vi "Пwiczenie 1.vi"() -> ()   [LabVIEW 2017]
panel:
  in  "Czyœæ":bool
  out "Aktualny wynik":dbl format="%#.1f"
  in  "Czêstotliwoœæ próbkowania":u16(ring) items=["1 Hz"=1, "2 Hz"=2, "5 Hz"=5, "10 Hz"=10]
  in  "Okres":dbl(knob) step=2.0 scale=0.0..60.0
  in  "Amplituda":dbl(knob) step=1.0 scale=0.0..100.0
  in  "Czas narastania":dbl(knob) step=1.0 scale=0.0..60.0
  in  "Amplituda":dbl(knob) step=1.0 scale=0.0..100.0
  in  "Max":dbl(knob) step=1.0 scale=0.0..100.0
  in  "Min":dbl(knob) max=30.0 step=1.0 scale=0.0..100.0
  out "Wynik":dbl(graph)
  in  "STOP":bool
  in  "Tryb pracy":i32(knob) scale=1.0..3.0
  # "TRYB 1 - WARTOŒCI LOSOWE"
  # "TRYB 2 - SYGNA£ PI£OKSZTA£TNY"
  # "TRYB  3 - SYGNA£ TRÓJK¥TNY"
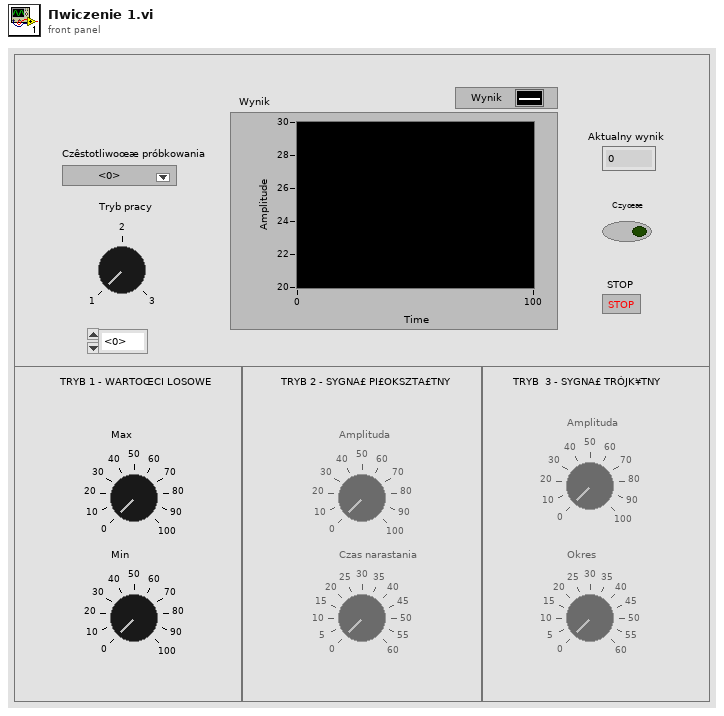
[diagram p1: front panel]
types:
  T1 = enum8{"Enabled", "Disabled", "Disabled and Grayed Out"}
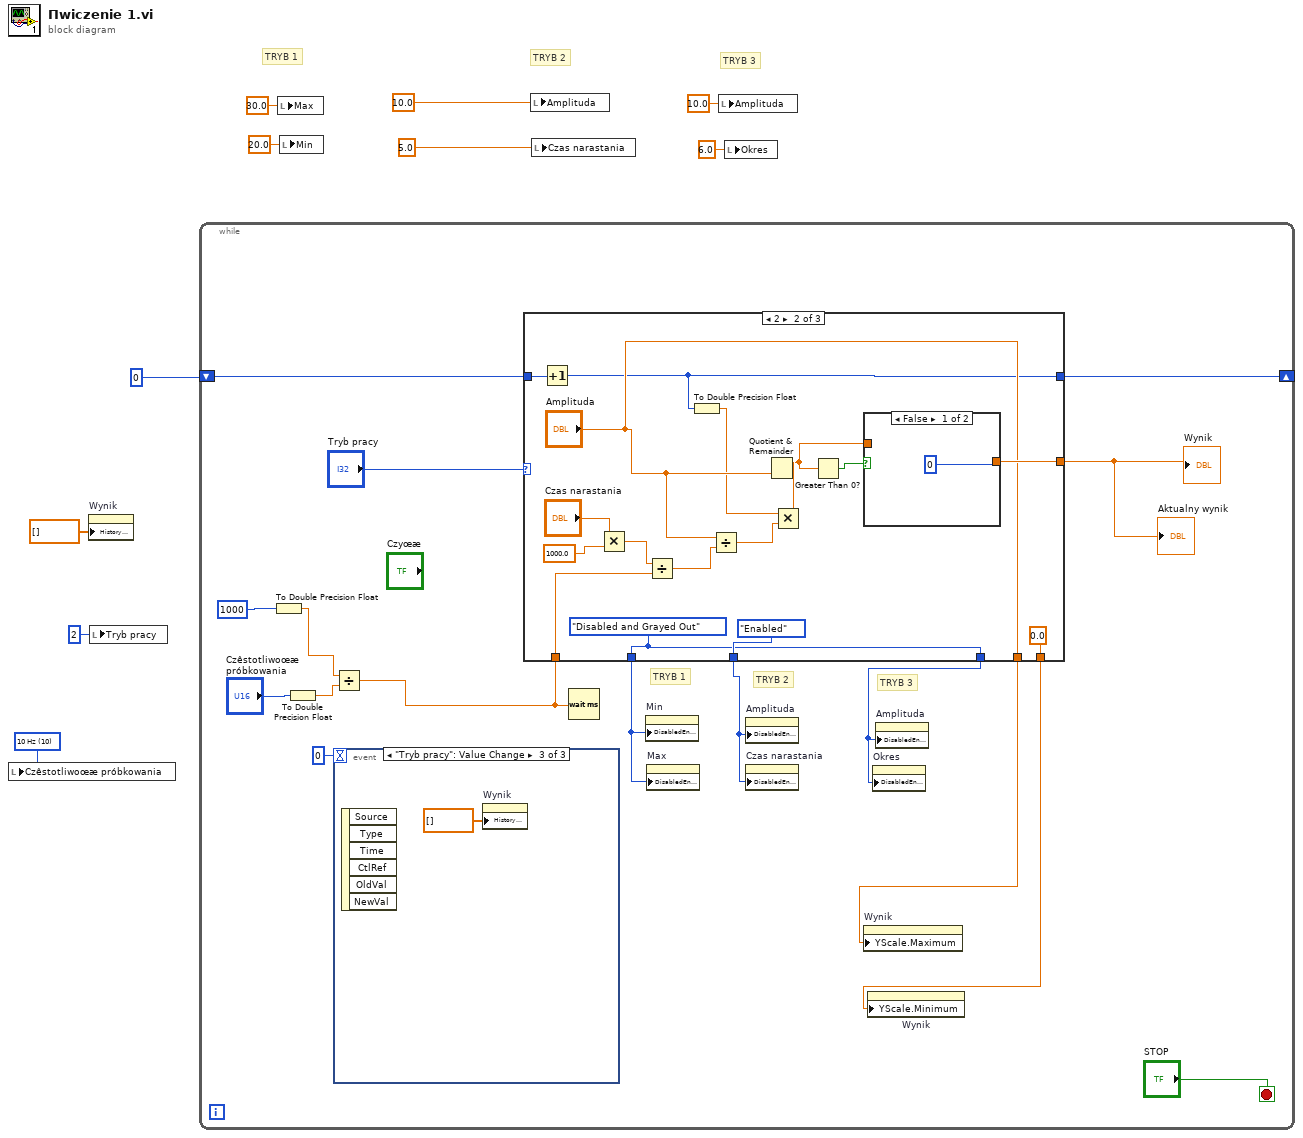
[diagram p0: block diagram]
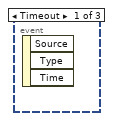
[diagram p2: hidden frame]
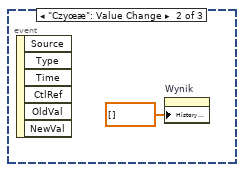
[diagram p3: hidden frame]
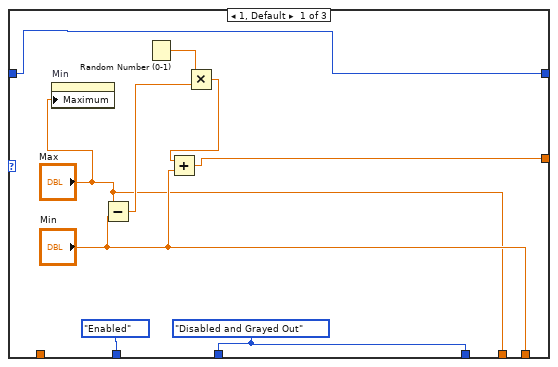
[diagram p4: hidden frame]
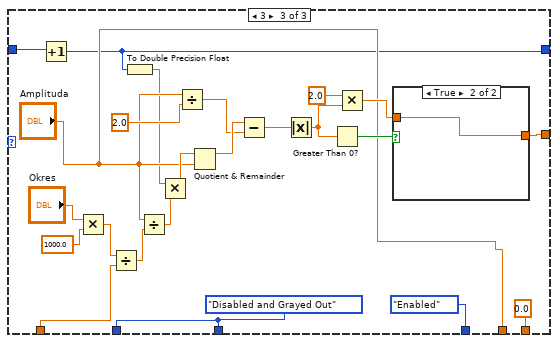
[diagram p6: hidden frame]
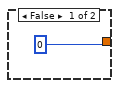
[diagram p7: hidden frame]
diagram:
  w9 = u16 10 items=["1 Hz"=1, "2 Hz"=2, "5 Hz"=5, "10 Hz"=10] ("Ring")
  # "TRYB 3"
  # "TRYB 2"
  # "TRYB 1"
  n1 = local write "Czêstotliwoœæ próbkowania"(w9) -> ()
  n2 = property on="Wynik" class="WFChart (strict)"("History Data"=dbl[] []) -> ()  [unwired: 2 in, 2 out]
  n3 = local write "Tryb pracy"(2 ("Tryb pracy")) -> ()
  n4 = while {
    shift-right: [w24] -> _
    shift-left: 0 -> [w23]
    stop <- "STOP" stop-if-true
    # "TRYB 3"
    # "TRYB 1"
    # "TRYB 2"
    n5 = To Double Precision Float(number=1000) -> (double precision float=w13:dbl)
    n6 = To Double Precision Float(number="Czêstotliwoœæ próbkowania") -> (double precision float=w11:dbl)
    n7 = Divide(x=w13, y=w11) -> (x/y=w19:dbl)
    n8 = event shown="[2] \"Tryb pracy\": Value Change" {
      selector: _ -> [_ _ _]
      dyn-events: _ -> [_ _ _]
      timeout: 0 -> [_ _ _]
      event Timeout {
        n9 = event-data() -> ()  [unwired: 1 in, 3 out]
      }
      event "Czyœæ": Value Change {
        n10 = event-data() -> ()  [unwired: 1 in, 6 out]
        n11 = property on="Wynik" class="WFChart (strict)"("History Data"=dbl[] []) -> ()  [unwired: 2 in, 2 out]
      }
      event "Tryb pracy": Value Change {
        n12 = event-data() -> ()  [unwired: 1 in, 6 out]
        n13 = property on="Wynik" class="WFChart (strict)"("History Data"=dbl[] []) -> ()  [unwired: 2 in, 2 out]
      }
    }
    n14 = case shown="2" "Tryb pracy" {
      tunnel: [w34 w44 w71] -> w18
      tunnel: [w33 w39 w58] -> w24
      tunnel: w23 -> [w33 w54 w72]
      tunnel: w19 -> [_ w50 w73]
      tunnel: [w31 T1."Enabled" ("Disabled") w65] -> w22
      tunnel: [T1."Enabled" ("Disabled") w42 w65] -> w21
      tunnel: [w31 w42 T1."Enabled" ("Disabled")] -> w20
      tunnel: ["Min" 0.0 ("Min") 0.0 ("Min")] -> w16
      tunnel: ["Max" "Amplituda" "Amplituda"] -> w15
      frame 1, Default {
        w31 = T1."Disabled and Grayed Out" ("Disabled")
        n15 = property on="Min" class="Knob (strict)"("Maximum"="Max") -> ()  [unwired: 2 in, 2 out]
        n16 = Subtract(x="Max", y="Min") -> (x-y=w36:dbl)
        n17 = Random Number (0-1)() -> (number: 0 to 1=w37:dbl)
        n18 = Multiply(x=w37, y=w36) -> (x*y=w35:dbl)
        n19 = Add(x=w35, y="Min") -> (x+y=w34:dbl)
      }
      frame 2 {
        w42 = T1."Disabled and Grayed Out" ("Disabled")
        n20 = Increment(x=w54) -> (x+1=w39:i32)
        n21 = Multiply(x="Czas narastania", y=1000.0) -> (x*y=w51:dbl)
        n22 = Divide(x=w51, y=w50) -> (x/y=w49:dbl)
        n23 = To Double Precision Float(number=w39) -> (double precision float=w38:dbl)
        n24 = Divide(x="Amplituda", y=w49) -> (x/y=w48:dbl)
        n25 = Multiply(x=w38, y=w48) -> (x*y=w47:dbl)
        n26 = Quotient & Remainder(x=w47, y="Amplituda") -> (x-y*floor(x/y)=w45:dbl)  [unwired: 1 out]
        n27 = Greater Than 0?(x=w45) -> (x > 0?=w46:bool)
        n28 = case shown="False" w46 {
          tunnel: w45 -> [_ w56]
          tunnel: [0 w56] -> w44
          frame False {
          }
          frame True {
          }
        }
      }
      frame 3 {
        w65 = T1."Disabled and Grayed Out" ("Disabled")
        n29 = Increment(x=w72) -> (x+1=w58:i32)
        n30 = Multiply(x="Okres", y=1000.0) -> (x*y=w78:dbl)
        n31 = Divide(x=w78, y=w73) -> (x/y=w77:dbl)
        n32 = To Double Precision Float(number=w58) -> (double precision float=w57:dbl)
        n33 = Divide(x="Amplituda", y=w77) -> (x/y=w76:dbl)
        n34 = Multiply(x=w57, y=w76) -> (x*y=w75:dbl)
        n35 = Divide(x="Amplituda", y=2.0) -> (x/y=w68:dbl)
        n36 = Quotient & Remainder(x=w75, y="Amplituda") -> (x-y*floor(x/y)=w69:dbl)  [unwired: 1 out]
        n37 = Subtract(x=w69, y=w68) -> (x-y=w67:dbl)
        n38 = Absolute Value(x=w67) -> (abs(x)=w63:dbl)
        n39 = Greater Than 0?(x=w63) -> (x > 0?=w66:bool)
        n40 = Multiply(x=2.0, y=w63) -> (x*y=w61:dbl)
        n41 = case shown="True" w66 {
          tunnel: w61 -> [_ w81]
          tunnel: [0 w81] -> w71
          frame False {
          }
          frame True {
          }
        }
      }
    }
    "Wynik" <- w18
    "Aktualny wynik" <- w18
    n42 = Wait (ms)(milliseconds to wait=w19) -> ()  [unwired: 1 out]
    n43 = property on="Min" class="Knob (strict)"("DisabledEnum"=w21) -> ()  [unwired: 2 in, 2 out]
    n44 = property on="Max" class="Knob (strict)"("DisabledEnum"=w21) -> ()  [unwired: 2 in, 2 out]
    n45 = property on="Amplituda" class="Knob (strict)"("DisabledEnum"=w22) -> ()  [unwired: 2 in, 2 out]
    n46 = property on="Czas narastania" class="Knob (strict)"("DisabledEnum"=w22) -> ()  [unwired: 2 in, 2 out]
    n47 = property on="Wynik" class="WFChart (strict)"("YScale.Maximum"=w15) -> ()  [unwired: 2 in, 2 out]
    n48 = property on="Wynik" class="WFChart (strict)"("YScale.Minimum"=w16) -> ()  [unwired: 2 in, 2 out]
    n49 = property on="Okres" class="Knob (strict)"("DisabledEnum"=w20) -> ()  [unwired: 2 in, 2 out]
    n50 = property on="Amplituda" class="Knob (strict)"("DisabledEnum"=w20) -> ()  [unwired: 2 in, 2 out]
  }
  n51 = local write "Max"(30.0 ("Max")) -> ()
  n52 = local write "Min"(20.0 ("Min")) -> ()
  n53 = local write "Amplituda"(10.0 ("Amplituda")) -> ()
  n54 = local write "Czas narastania"(5.0 ("Czas narastania")) -> ()
  n55 = local write "Amplituda"(10.0 ("Amplituda")) -> ()
  n56 = local write "Okres"(6.0 ("Okres")) -> ()
